vi "Async Tx Cyclic Engine.vi"(7 "error in (no error)":errorcluster, 10 "Tx Cyclic Async":T1) -> (0 "error out":errorcluster)   [LabVIEW 2020, in "985x Support Addon Engine.lvlib"]
uses:
  985x Support Addon Engine.lvlib
  <vilib>/platform/TimedLoop/XDataNode/XDataNode.xnode
  <vilib>/Platform/TimedLoop/XDataNode/nitl_modes.ctl
  <vilib>/Platform/TimedLoop/XDataNode/XDNodeRunTimeDep.lvlib
  <vilib>/Platform/TimedLoop/XDataNode/wakeup.ctl
  <vilib>/Platform/TimedLoop/XDataNode/timing_clust.ctl
  <vilib>/xnet/xnet.llb/XNET Convert (Signal to Frame CAN).vi
  Types/Cyclic Frame Info.ctl
  Types/FPGA Refnum.ctl
  Types/Tx Cyclic Async Info.ctl
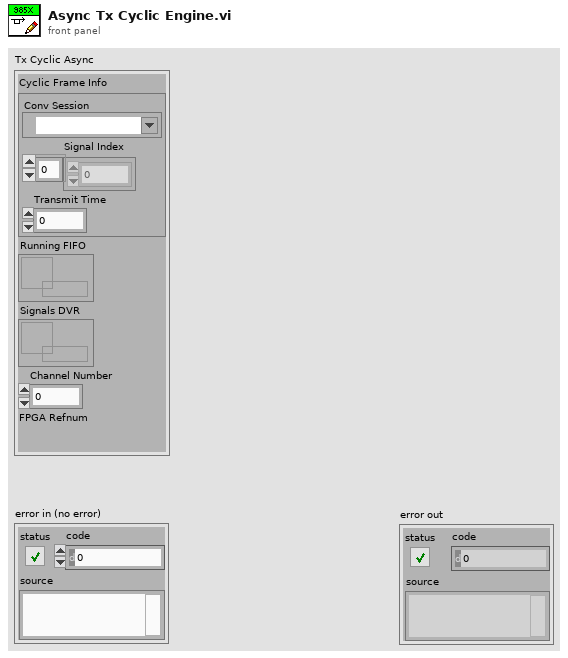
[diagram p1: front panel]
types:
  T1 = typedef "985x Support Addon Engine.lvlib/Tx Cyclic Async Info.ctl" = cluster{"Cyclic Frame Info":T2, "Running FIFO":refnum<k33>, "Signals DVR":refnum<data-value>, "Channel Number":u32, "FPGA Refnum":T3}
  T2 = typedef "985x Support Addon Engine.lvlib/Cyclic Frame Info.ctl" = cluster{"Conv Session":refnum<k21>, "Signal Index":u32[], "Transmit Time":dbl}
  T3 = typedef "985x Support Addon Engine.lvlib/FPGA Refnum.ctl" = refnum<k20>
  T4 = typedef "XDNodeRunTimeDep.lvlib/timing_clust.ctl" = cluster{"Expected End [f-1]":u64, "Actual End [f-1]":u64, "Finished Late? [f-1]":bool, "Expected End [i-1]":u64, "Actual End [i-1]":u64, "Finished Late? [i-1]":bool, "Expected Start [i]":u64, "Actual Start [i]":u64, "Expected Start [f]":u64, "Actual Start [f]":u64, "Source Name":string, "Structure Name":string, "Period":i64, "Deadline":i64, "Offset":i64, "Start":i64, "Priority":i32, "Timeout":i32, "Mode":T5, "Wakeup Reason":T6, "Error":errorcluster, "Source Type":string, "Secondary Source Type":string, "Global End Time":u64, "Global Start Time":u64, "Frame Duration":u64, "Iteration Duration":u64, "Assigned CPU":i32, "I/O Scan Engine Mode":u32}
  T5 = typedef "XDNodeRunTimeDep.lvlib/nitl_modes.ctl" = enum32{"No Change", "Process missed periods, maintain original phase", "Discard missed periods, maintain original phase", "Process missed periods, ignore original phase", "Discard missed periods, ignore original phase"}
  T6 = typedef "XDNodeRunTimeDep.lvlib/wakeup.ctl" = enum32{"Normal", "Aborted", "Asynchronous wakeup", "Timing source error", "Timed loop error", "Timeout"}
  T7 = typedef "XNET Frame CAN.ctl" = cluster{"timestamp":timestamp, "payload":u8[], "identifier":u32, "type":T8, "extended?":bool, "echo?":bool}
  T8 = typedef "XNET Frame Type CAN.ctl" = u8
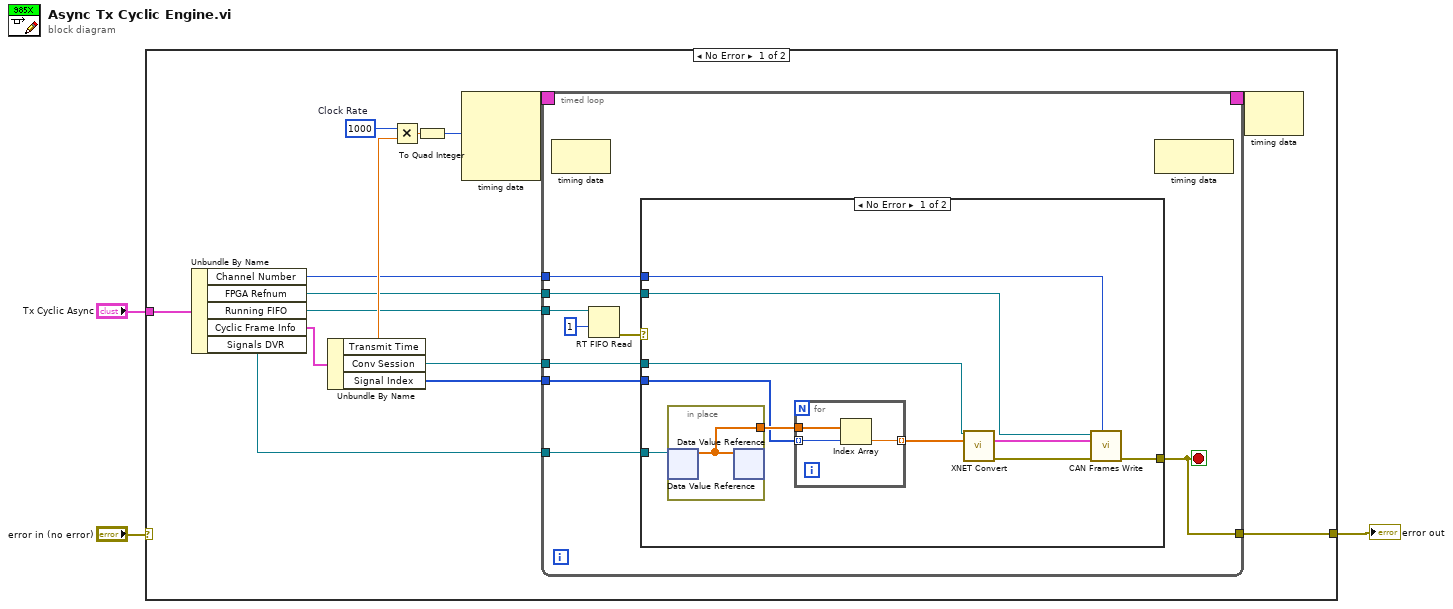
[diagram p0: block diagram]
diagram:
  n1 = case shown="No Error" "error in (no error)" {
    selector: "error in (no error)" -> [_ w49]
    tunnel: [w10 w49] -> w2
    tunnel: "Tx Cyclic Async" -> [w9 _]
    frame No Error {
      w15 = i64 1000  # Clock Rate
      n2 = Unbundle By Name(w9) -> ("Channel Number"=w6:u32, "FPGA Refnum"=w4:T3, "Running FIFO"=w7:refnum<k33>, "Cyclic Frame Info"=w8:T2, "Signals DVR"=w5:refnum<data-value>)
      n3 = Unbundle By Name(w8) -> ("Transmit Time"=w16:dbl, "Conv Session"=w12:refnum<k21>, "Signal Index"=w11:u32[])
      n4 = Multiply(x=w15, y=w16) -> (x*y=w14:dbl)
      n5 = To Quad Integer(1:w14) -> (0:w13:i64)
      n6 = node-c288(w13) -> (w18:T4)  [unwired: 3 in]
      n7 = timed-loop {
        timing: w18 -> [_]
        timing-out: [_] -> w17
        tunnel: w7 -> [w26]
        tunnel: w12 -> [w24]
        tunnel: w11 -> [w23]
        tunnel: w5 -> [w22]
        tunnel: w6 -> [w21]
        tunnel: [w20] -> w10
        tunnel: w4 -> [w19]
        stop <- w20 stop-if-true
        n8 = node-c288() -> ()  [unwired: 1 in, 1 out]
        n9 = RT FIFO Read(0:w26, 2:1 ("timeout in ms (0)")) -> (11:w25:errorcluster)  [unwired: 2 in, 4 out]
        n10 = case shown="No Error" w25 {
          selector: w25 -> [_ w44]
          tunnel: w24 -> [w36 _]
          tunnel: w23 -> [w37 _]
          tunnel: w22 -> [w39 _]
          tunnel: w21 -> [w33 _]
          tunnel: [w31 w44] -> w20
          tunnel: w19 -> [w30 _]
          frame No Error {
            n11 = in-place {
              in-place-border: [w40] -> w38
              n12 = in-place-dvr #1(w39) -> (w40:dbl[])  [unwired: 1 out]
              n13 = in-place-dvr #1(w40) -> ()  [unwired: 2 out]
            }
            n14 = for {
              tunnel: w38 -> [w43]
              tunnel: w37 -> [w42] mode=indexing
              tunnel: [w41] -> w35 mode=indexing
              n15 = Index Array(array=w43, index=w42) -> (element=w41:dbl)
            }
            n16 = call-poly <vilib>:"XNET Convert.vi"("session in"=w36, "signal data"=w35) -> ("frame data"=w34:T7[], "error out"=w32:errorcluster)  [unwired: 1 in, 11 out]
            n17 = call "CAN Frames Write.vi"("Channel Number"=w33, "error in (no error)"=w32, "Frames"=w34, "FPGA Refnum"=w30) -> ("error out"=w31:errorcluster)  [unwired: 7 in]
          }
          frame Error {
          }
        }
        n18 = node-c288() -> ()  [unwired: 1 in, 1 out]
      }
      n19 = node-c288(w17) -> ()  [unwired: 1 out]
    }
    frame Error {
    }
  }
  "error out" <- w2
